vi "change freq.vi"() -> ()   [LabVIEW 2016]
panel:
  out "Status OUT":T1
  out "error out":errorcluster
  in  "error in":errorcluster={"status"=FALSE, "code"=0, "source"="OK"}
  in  "m/c temp setpoint":dbl=50.0 format="%#_13g"
  in  "function":enum16{"Ramp", "Triangle", "Sine"}(ring)
  in  "phase":dbl
  in  "cycles (1,2,...)":i32=1 min=1 step=1
  in  "step size":dbl=500.0 format="%.4f"
  in  "Min":dbl=500.0
  in  "Max":dbl=5000.0
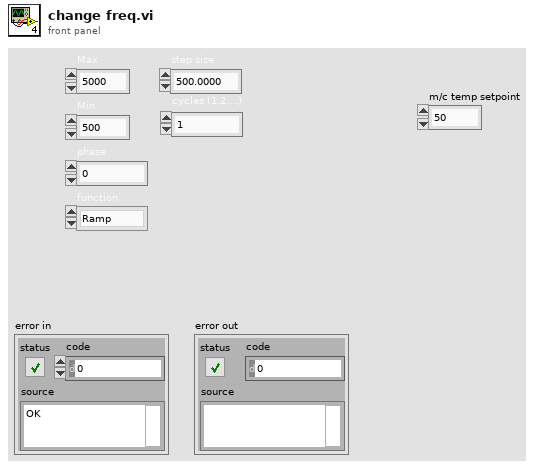
[diagram p1: front panel]
types:
  T1 = cluster{"axis 1: Current position (°)":dbl, "axis 2: Current position (°)":dbl, "axis 1: rot. count":dbl, "axis 2: rot. count":dbl, "axis 1: StepWidth":dbl, "axis 2: StepWidth":dbl, "axis 1: speed (°/s)":dbl, "axis 2: speed (°/s)":dbl, "axis 1: positioner status":cluster{"moving":bool, "stop detected":bool, "sensor error":bool, "sensor disconnected":bool}, "axis 2: positioner status":cluster{"moving":bool, "stop detected":bool, "sensor error":bool, "sensor disconnected":bool}}
  T2 = cluster{"axis 1: Amplitude [V]":dbl, "axis 2: Amplitude [V]":dbl, "axis 1: DCLevel [V]":dbl, "axis 2: DCLevel [V]":dbl, "axis 1: Frequency [Hz]":dbl, "axis 2: Frequency [Hz]":dbl, "axis 1: sp position °":dbl, "axis 2: sp position °":dbl, "axis 1: sp rot count":dbl, "axis 2: sp rot count":dbl}
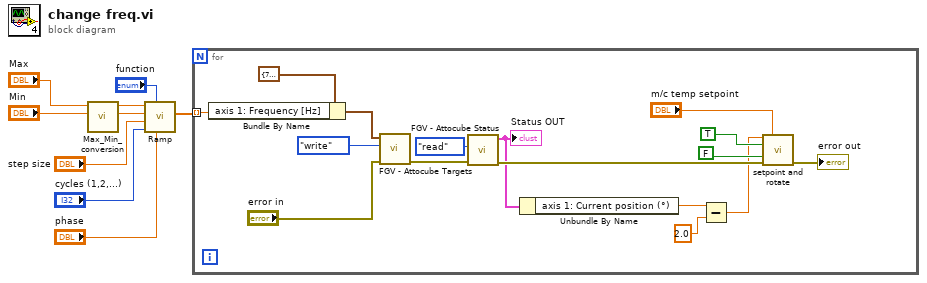
[diagram p0: block diagram]
diagram:
  n1 = call <userlib>:"Max_Min_conversion.vi"("Min"="Min", "Max"="Max") -> ("offset"=w8:dbl, "Amplitude"=w9:dbl)  [unwired: 8 in]
  n2 = call <userlib>:"Ramp.vi"("phase"="phase", "function (ramp)"="function", "cycles (1,2,...)"="cycles (1,2,...)", "step size"="step size", "offset"=w8, "amplitude"=w9) -> ("Waveform Graph"=w1:dbl[])  [unwired: 3 in, 2 out]
  n3 = for {
    tunnel: w1 -> [w23] mode=indexing
    n4 = Bundle By Name(cluster=T2 {"axis 1: Amplitude [V]"=70.0, "axis 2: Amplitude [V]"=0.0, "axis 1: DCLevel [V]"=0.0, "axis 2: DCLevel [V]"=0.0, "axis 1: Frequency [Hz]"=3000.0, "axis 2: Frequency [Hz]"=3000.0, "axis 1: sp position °"=250.0, "axis 2: sp position °"=255.0, "axis 1: sp rot count"=0.0, "axis 2: sp rot count"=0.0} ("Targets In"), "axis 1: Frequency [Hz]"=w23) -> (w22:T2)
    n5 = call "FGV - Attocube Targets.vi"("error in"="error in", "Function"=enum16{"write", "read"}."write", "Targets In"=w22) -> ("error out"=w19:errorcluster)  [unwired: 3 in, 1 out]
    n6 = call "FGV - Attocube Status.vi"("error in"=w19, "Function"=enum16{"write", "read"}."read") -> ("error out"=w18:errorcluster, "Status OUT"=w15:T1)  [unwired: 4 in]
    "Status OUT" <- w15
    n7 = Unbundle By Name(w15) -> ("axis 1: Current position (°)"=w12:dbl)
    n8 = Subtract(x=w12, y=2.0) -> (x-y=w10:dbl)
    n9 = call "setpoint and rotate.vi"("axis 1: sp position °"=w10, "m/c temp setpoint"="m/c temp setpoint", "move axis 1"=TRUE, "move axis 2"=FALSE, "error in"=w18) -> ("error out"=→"error out":errorcluster)  [unwired: 9 in, 1 out]
  }
